vi "InnerCallbackOnWriteTree.vi"(8 "error in":errorcluster, 10 "node (for type)":refnum<class "control module editor.lvclass">, 11 "node reference":refnum<data-value>) -> (0 "error out":errorcluster)   [LabVIEW 2013, in "control module editor.lvclass"]
uses:
  control module editor.lvclass
  <vilib>/NI/Configuration Framework/Node/NISE_CEF_Node.lvclass
  configuration/control module configuration.lvclass
  <vilib>/NI/Configuration Framework/serializable configuration/NISE_CEF_serializable configuration.lvclass/NISE_CEF_serializable configuration.ctl
  <vilib>/NI/Configuration Framework/serializable configuration/Read UID.vi
  read fixed channel configuration.vi
  <vilib>/Utility/LVClass/Get LV Class Name.vi
  <vilib>/NI/Configuration Framework/error generator/NISE_error generator.vi
  Configuration Editor/Classes/Engine Parent/Engine Parent Editor Node.lvclass
  <vilib>/NI/Module Execution Interface/Engine Configuration/engine configuration.lvclass
  Configuration Editor/Classes/Module editor node/module editor node.lvclass
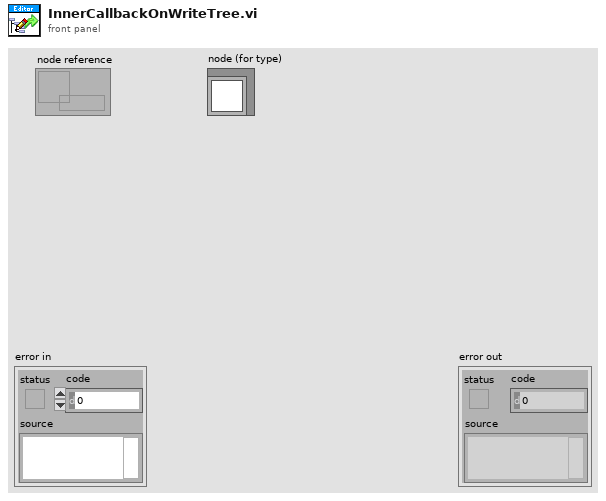
[diagram p1: front panel]
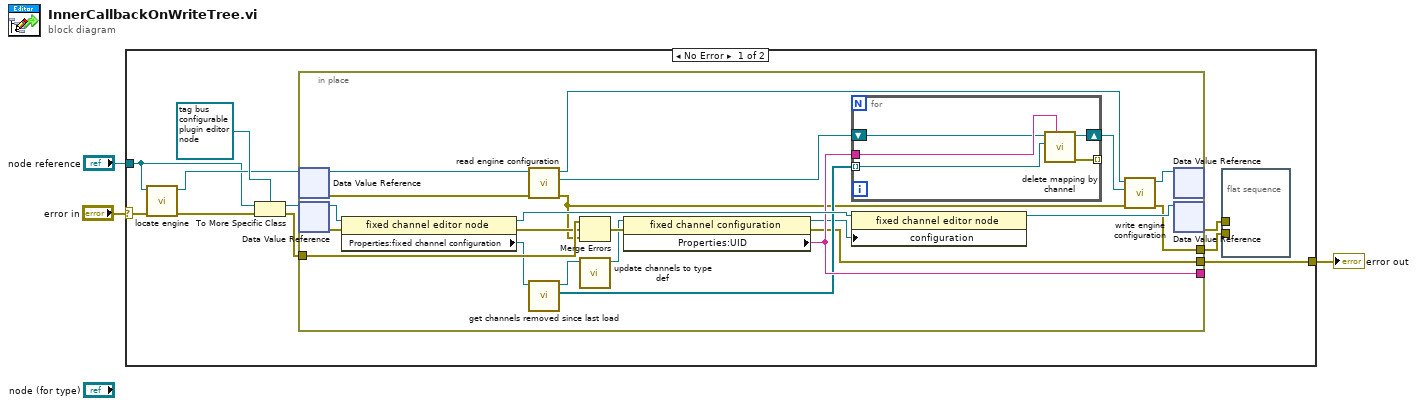
[diagram p0: block diagram]
diagram:
  n1 = case shown="No Error" "error in" {
    selector: "error in" -> [w4 w41]
    tunnel: "node reference" -> [w8 _]
    tunnel: [w7 w41] -> w2
    frame No Error {
      n2 = call "locate engine.vi"("error in"=w4, "component"=w8) -> ("error out"=w9:errorcluster, "engine"=w10:refnum<data-value>)  [unwired: 8 in]
      n3 = To More Specific Class(target class=refnum<data-value> refnum ("data value reference"), reference=w8, error in=w9) -> (specific class reference=w12:refnum<data-value>, error out=w11:errorcluster)
      n4 = in-place {
        in-place-border: w11 -> [w35]
        in-place-border: [w25] -> w7
        in-place-border: [w27] -> _
        in-place-border: [w18] -> w5
        n5 = in-place-dvr #1(w10) -> (w34:refnum<class "Engine Parent Editor Node.lvclass">, w30:errorcluster)
        n6 = in-place-dvr #2(w12) -> (w32:refnum<class "control module editor.lvclass">, w28:errorcluster)
        n7 = property class="fixed channel editor node"(reference=w32, error in=w28) -> (reference out=w29:refnum<class "control module editor.lvclass">, error out=w24:errorcluster, "Properties:fixed channel configuration"=w16:refnum<class "control module configuration.lvclass">)
        n8 = call "read engine configuration.vi"("error in"=w30, "Engine Parent Editor Node in"=w34) -> ("error out"=w19:errorcluster, "engine configuration"=w14:refnum<class "engine configuration.lvclass">, "Engine Parent Editor Node out"=w33:refnum<class "Engine Parent Editor Node.lvclass">)  [unwired: 7 in]
        n9 = call "get channels removed since last load.vi"("fixed channel configuration in"=w16) -> ("removed"=w26:refnum<class "TBM channel.lvclass">[], "fixed channel configuration out"=w22:refnum<class "control module configuration.lvclass">)  [unwired: 9 in]
        n10 = Merge Errors(w35, w24, w19) -> (w31:errorcluster)
        n11 = call-dynamic "update channels to type def.vi"("fixed channel configuration in"=w22) -> ("fixed channel configuration out"=w21:refnum<class "control module configuration.lvclass">)  [unwired: 10 in]
        n12 = property class="fixed channel configuration"(reference=w21, error in=w31) -> (reference out=w17:refnum<class "control module configuration.lvclass">, error out=w25:errorcluster, "Properties:UID"=w27:string)
        n13 = for {
          tunnel: w27 -> [w40]
          tunnel: w26 -> [w39] mode=indexing
          shift-right: [w38] -> w15
          shift-left: w14 -> [w37]
          tunnel: [w36] -> _ mode=indexing
          n14 = call <vilib>:"delete mapping by channel.vi"("owner ID"=w40, "channel"=w39, "engine configuration in"=w37) -> ("error out"=w36:errorcluster, "engine configuration out"=w38:refnum<class "engine configuration.lvclass">)  [unwired: 7 in]
        }
        n15 = property class="fixed channel editor node"(reference=w29, "configuration"=w17) -> (reference out=w23:refnum<class "control module editor.lvclass">)  [unwired: 1 in, 1 out]
        n16 = call "write engine configuration.vi"("error in"=w19, "engine configuration"=w15, "Engine Parent Editor Node in"=w33) -> ("error out"=w18:errorcluster, "Engine Parent Editor Node out"=w20:refnum<class "Engine Parent Editor Node.lvclass">)  [unwired: 7 in]
        n17 = in-place-dvr #1(w20) -> ()  [unwired: 2 out]
        n18 = in-place-dvr #2(w23) -> (w6:errorcluster)  [unwired: 1 out]
      }
      n19 = flat-sequence {
        tunnel: w6 -> [_]
        tunnel: w5 -> [_]
        frame #0 {
        }
      }
    }
    frame Error {
    }
  }
  "error out" <- w2
